vi "Periodic Tasks.vi"(8 "error in":errorcluster) -> ()   [LabVIEW 2014]
doc: "This VI runs in parallel to other tasks. It can contain as many user-defined periodic loops as you need. These can carry out PID or other sorts of timed response."
uses:
  NavX/navX-MXP Library/COMMON/TypeDefs/navX YPRH Data.ctl
  <vilib>/Rock Robotics/WPI/DriverStation/WPI_DriverStationRobotMode2.ctl
  <vilib>/Rock Robotics/WPI/Solenoid/WPI_SolenoidValue.ctl
  <vilib>/Rock Robotics/WPI/RobotDrive/WPI_RobotDriveGetSetRefNum.vi
  Robot Global Data.vi
  <vilib>/addons/control/pid/pid.llb/PID (DBL).vi
  <vilib>/Rock Robotics/WPI/RobotDrive/WPI_RobotDriveMecanumDrive_Cartesian.vi
  <vilib>/Rock Robotics/Network Tables/SD Write Numeric Array.vi
  <vilib>/Rock Robotics/Network Tables/SD Write Number.vi
  <vilib>/Rock Robotics/WPI/Joystick/WPI_JoystickGetSetRefNum.vi
  <vilib>/Rock Robotics/Network Tables/SD Write Boolean.vi
  <vilib>/Rock Robotics/Network Tables/SD Write String.vi
  <vilib>/Rock Robotics/WPI/Solenoid/WPI_SolenoidSetEnum.vi
  <vilib>/Rock Robotics/Network Tables/SD Read String.vi
  <vilib>/Utility/file.llb/Write To Spreadsheet File (DBL).vi
  <vilib>/addons/control/pid/pid.llb/PID Output Rate Limiter (DBL).vi
  NavX/navX-MXP Library/navX-MXP IMU.lvlib
  <vilib>/addons/control/pid/NI_PID_pid.lvlib
panel:
  in  "Turn PID Gains(Teley)":T1={"proportional gain (Kc)"=0.02, "integral time (Ti, min)"=0.0, "derivative time (Td, min)"=0.0}
  out "Angle":dbl
  out "Elevator Setpoint Limited":dbl
  out "Angle Data":T2(graph)
  in  "Manual Rate":dbl=30.0
  in  "Elevator PID gains (Seperation Corector)":T1={"proportional gain (Kc)"=0.007, "integral time (Ti, min)"=0.0, "derivative time (Td, min)"=0.0} {"derivative time (Td, min)" format="%.3f"; "integral time (Ti, min)" format="%.3f"; "proportional gain (Kc)" format="%.3f"}
  in  "Elevator Output Range (Seperation Corector)":cluster{"output high":dbl, "output low":dbl}={"output high"=0.25, "output low"=-0.1} {"output low" format="%.2f"; "output high" format="%.2f"}
  out "Encoder Ticks":i16
  in  "Elevator Output Range (RLPC/AVG)":cluster{"output high":dbl, "output low":dbl}={"output high"=1.0, "output low"=-0.5}
  out "Elevator Currents (A)":cluster{"current (A)":dbl, "current (A)":dbl}(graph)
  in  "output rate (EGU/min)":dbl=100000.0 format="%.2f"
  in  "Spin Cutoff":dbl=2.0
  in  "Elevator Cutoff Pos":dbl=20.0
  in  "Elevator PID Gains (RLPC/AVG)":T1={"proportional gain (Kc)"=0.003, "integral time (Ti, min)"=0.0, "derivative time (Td, min)"=0.0} {"proportional gain (Kc)" min=0.0 step=0.05 format="%.3f"; "integral time (Ti, min)" step=0.005 format="%.3f"; "derivative time (Td, min)" format="%.3f"}
  out "Elevator Setpoint":dbl
  in  "Turn PID Gains(Auto)":T1={"proportional gain (Kc)"=0.01, "integral time (Ti, min)"=0.016, "derivative time (Td, min)"=0.0} {"derivative time (Td, min)" format="%.3f"; "integral time (Ti, min)" format="%.3f"; "proportional gain (Kc)" format="%.3f"}
  out "Base PID Gains":T1={"proportional gain (Kc)"=1.0, "integral time (Ti, min)"=0.01, "derivative time (Td, min)"=0.0} {"derivative time (Td, min)" format="%.3f"; "integral time (Ti, min)" format="%.3f"; "proportional gain (Kc)" format="%.3f"}
  out "Spin Joy X":dbl
  in  "Use Knob?":bool=TRUE
  out "error out":errorcluster
  out "Y Setpoint":dbl
  out "X Setpoint":dbl
  out "Elevator Data":T3(graph)
  out "Closed Loop":bool
  out "Rear Right Distance":dbl
  out "Rear Left Distance":dbl
  out "Front Right Distance":dbl
  out "Front Left Distance":dbl
  out "Rear Right Rate":dbl(knob) scale=-1.0..1.0
  out "Rear Left Rate":dbl(knob) scale=-1.0..1.0
  out "Front Right Rate":dbl(knob) scale=-1.0..1.0
  out "Front Left Rate":dbl(knob) scale=-1.0..1.0
  out "appended array":dbl[](array[numeric])
  out "Angular Target":dbl
  out "YPRH":T4
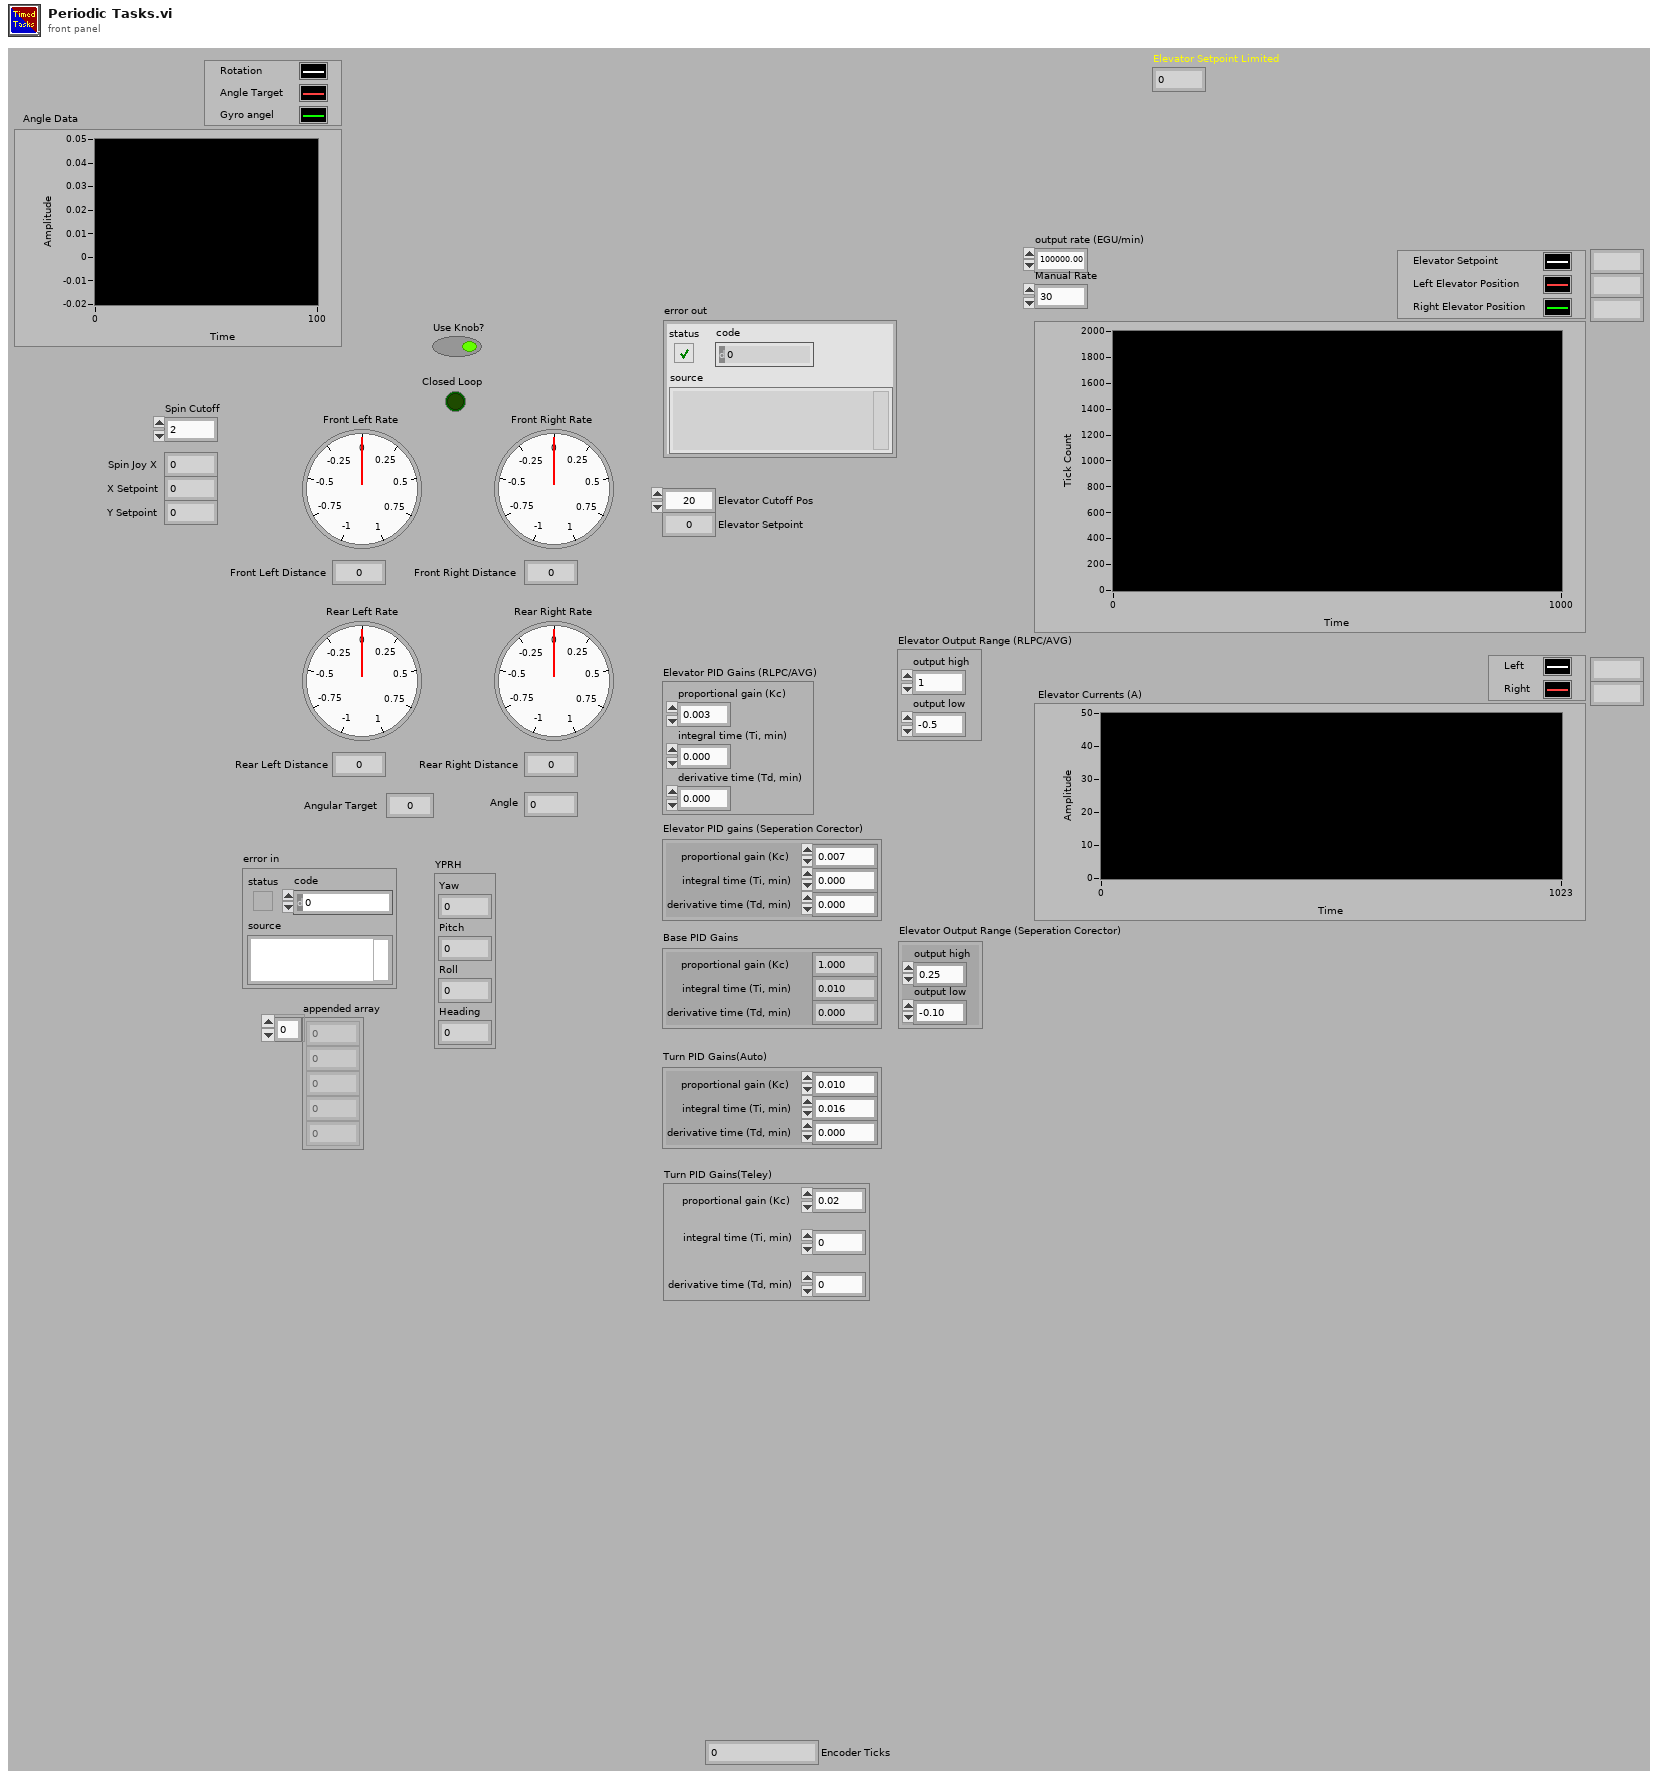
[diagram p1: front panel]
types:
  T1 = cluster{"proportional gain (Kc)":dbl, "integral time (Ti, min)":dbl, "derivative time (Td, min)":dbl}
  T2 = cluster{"t":dbl, "Angular Target":dbl, "Gyro Angle":dbl}
  T3 = cluster{"Elevator Setpoint":dbl, "Distance":dbl, "Distance":dbl}
  T4 = typedef "navX-MXP IMU.lvlib/navX YPRH Data.ctl" = cluster{"Yaw":dbl, "Pitch":dbl, "Roll":dbl, "Heading":dbl}
  T5 = typedef "WPI_EncoderDevRef.ctl" = cluster{"DevStatus":errorcluster, "EncoderIndex":T6, "CounterIndex":T7, "DistancePerCount":dbl, "Decoding Type":T8}
  T6 = typedef "FPGA_EncoderIdx.ctl" = enum8{"Enc 0", "Enc 1", "Enc 2", "Enc 3", "Enc 4", "Enc 5", "Enc 6", "Enc 7", "Invalid"}
  T7 = typedef "FPGA_CounterCtrSystemIndex.ctl" = enum8{"Ctr 0", "Ctr 1", "Ctr 2", "Ctr 3", "Ctr 4", "Ctr 5", "Ctr 6", "Ctr 7", "Invalid"}
  T8 = typedef "WPI_EncoderType.ctl" = enum16{"1x", "2x", "4x"}
  T9 = typedef "WPI_MotorControlDeviceRef.ctl" = cluster{"DeviceStatus":errorcluster, "Type":T10, "PWM":cluster{"Controller":T11, "PWM Channel":T12, "DeadBand":T13}, "CAN":cluster{"Device Number":u8, "Control Mode":T14, "Semaphore":T15, "Max Vout":dbl, "TalonSRX Control Mode":T16}, "Invert":bool, "TransformRef":T17, "InvTransformRef":T17}
  T10 = typedef "WPI_MotorControlType.ctl" = enum16{"PWM", "CAN", "CANTalonSRX"}
  T11 = typedef "FPGA_TypedefDigitalModule.ctl" = enum16{"Controller 1"}
  T12 = typedef "FPGA_DIOPWMChannel.ctl" = enum8{"PWM 0", "PWM 1", "PWM 2", "PWM 3", "PWM 4", "PWM 5", "PWM 6", "PWM 7", "PWM 8", "PWM 9", "PWM MXP 0", "PWM MXP 1", "PWM MXP 2", "PWM MXP 3", "PWM MXP 4", "PWM MXP 5", "PWM MXP 6", "PWM MXP 7", "PWM MXP 8", "PWM MXP 9", "Invalid"}
  T13 = typedef "WPI_PWMDeadband.ctl" = cluster{"Name":string, "maxPositivePwm":i32, "minPositivePwm":i32, "centerPwm":i32, "maxNegativePwm":i32, "minNegativePwm":i32, "angularRange":u16}
  T14 = typedef "WPI_CANJaguar_ControlMode.ctl" = enum8{"Percent VBus", "Current", "Speed", "Position", "Voltage"}
  T15 = typedef "Semaphore RefNum" = refnum<k1>
  T16 = typedef "WPI_CANTalonSRX_APIControlMode.ctl" = enum8{"Percent VBus", "Speed", "Position", "Slave", "Unchanged / Invalid"}
  T17 = typedef "WPI_PWMTransform_ConPane.ctl" = refnum<vi>
  T18 = typedef "WPI_DriverStationRobotMode2.ctl" = enum16{"Autonomous Disabled", "Autonomous Enabled", "Teleop Disabled", "Teleop Enabled", "Disconnected", "Finish", "Test Disabled", "Test Enabled", "Emergency Stopped"}
  T19 = cluster{"Elevator Setpoint Limited":dbl, "Distance":dbl, "Distance":dbl}
  T20 = typedef "navX-MXP IMU.lvlib/navX SPI DevRef.ctl" = cluster{"SPIDevRef":T21, "Board Information":T23, "Status":T24, "Offsets":cluster{"Yaw":dbl, "Quat W":dbl, "Quat X":dbl, "Quat Y":dbl, "Quat Z":dbl}, "Update Rate (4Hz-60Hz)":u8, "refnum name":string, "error":errorcluster}
  T21 = typedef "WPI_SPIDevRef.ctl" = cluster{"DevStatus":errorcluster, "Handle":i32, "Controller":T11, "SPI Bus":T22}
  T22 = typedef "spi_bus.ctl" = enum16{"SPI On-Board, CS0", "SPI On-Board, CS1", "SPI On-Board, CS2", "SPI On-Board, CS3", "SPI MXP", "Invalid"}
  T23 = typedef "navX-MXP IMU.lvlib/navX Board Information.ctl" = cluster{"WhoAmI (50 | 0x32)":u8, "Board Revision":u8, "Firmware Major Version":u8, "Firmware Minor Version":u8}
  T24 = typedef "navX-MXP IMU.lvlib/navX Status Data.ctl" = cluster{"Update Rate Hz":u8, "Accelerometer Full-Scale Range":u8, "Gyro Full-Scale Range":u16, "NAVX_OP_STATUS":T25, "NAVX_CAL_STATUS":T26, "NAVX_SELFTEST_STATUS":u8, "NAVX_SENSOR_STATUS":T27}
  T25 = typedef "navX-MXP IMU.lvlib/navX NAVX_OP_STATUS.ctl" = u8
  T26 = typedef "navX-MXP IMU.lvlib/navX NAVX_CAL_STATUS.ctl" = u8
  T27 = typedef "navX-MXP IMU.lvlib/navX NAVX_SENSOR_STATUS.ctl" = cluster{"MOVING":bool, "YAW_STABLE":bool, "MAG_DISTURBANCE":bool, "ALTITUDE_VALID":bool, "SEALEVEL_PRESS_SET":bool, "FUSED_HEADING_VALID":bool}
  T28 = typedef "WPI_RobotDriveDevRef.ctl" = cluster{"DevStatus":errorcluster, "Motors[]":T9[], "Square Inputs":bool, "Max Output":dbl}
  T29 = typedef "WPI_GyroDevRef.ctl" = cluster{"DevStatus":errorcluster, "Analog Module":T30, "Analog Channel":T31, "Offset":dbl, "Gain (VoltsPerDegree/Second)":dbl}
  T30 = typedef "FPGA_TypedefAnalogModule.ctl" = enum16{"Controller 1"}
  T31 = typedef "FPGA_AIChannel.ctl" = enum8{"AI 0", "AI 1", "AI 2", "AI 3", "AI MXP 0", "AI MXP 1", "AI MXP 2", "AI MXP 3", "Invalid"}
  T32 = typedef "WPI_SolenoidDevRef.ctl" = cluster{"DevStatus":errorcluster, "Pneumatics Control Module":u8, "Forward Solenoid Channel":T33, "Reverse Solenoid Channel":T33}
  T33 = typedef "WPI_SolenoidChannel.ctl" = enum8{"Solenoid 0", "Solenoid 1", "Solenoid 2", "Solenoid 3", "Solenoid 4", "Solenoid 5", "Solenoid 6", "Solenoid 7", "Invalid"}
  T34 = typedef "WPI_JoystickDevRef.ctl" = cluster{"Device":T35}
  T35 = typedef "WPI_JoystickDeviceEnum.ctl" = enum16{"USB 0", "USB 1", "USB 2", "USB 3", "USB 4", "USB 5"}
  T36 = typedef "WPI_SolenoidValue.ctl" = enum16{"Off", "On", "Forward", "Reverse"}
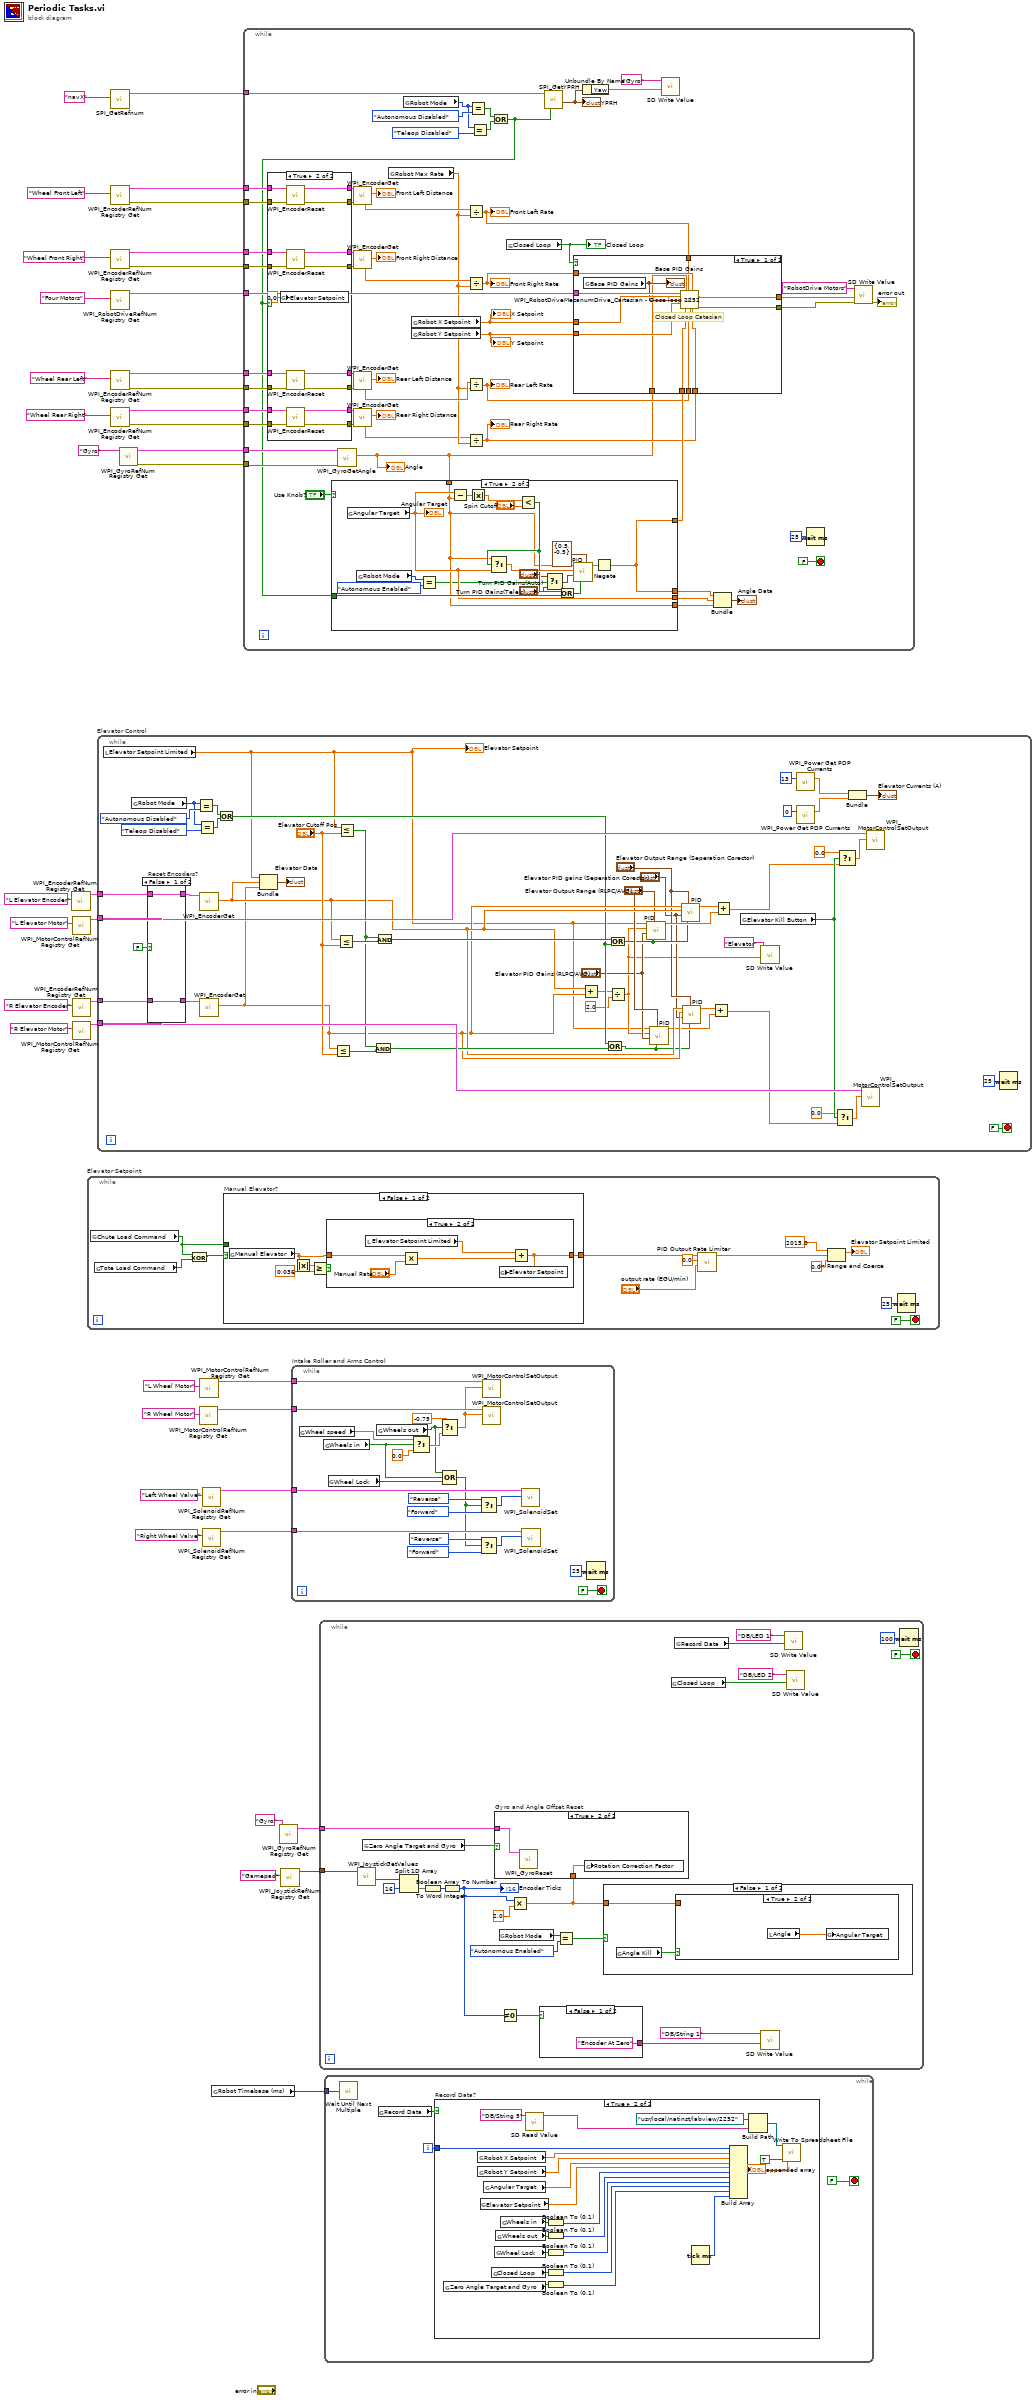
[diagram p0: block diagram]
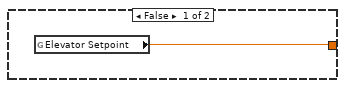
[diagram p2: hidden frame]
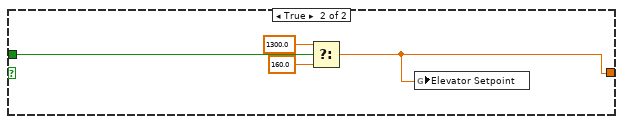
[diagram p3: hidden frame]
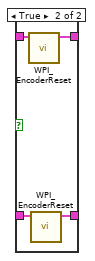
[diagram p4: hidden frame]
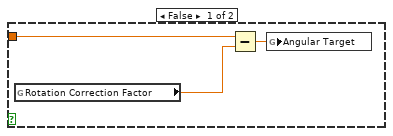
[diagram p5: hidden frame]
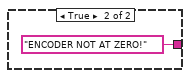
[diagram p7: hidden frame]
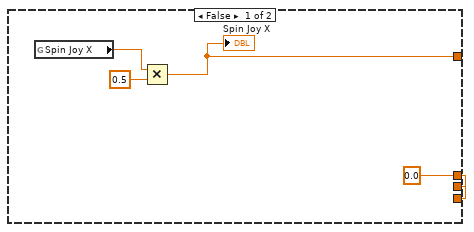
[diagram p11: hidden frame]
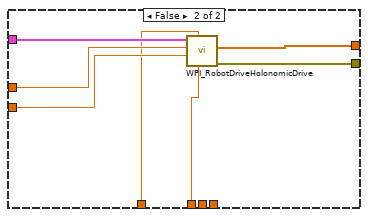
[diagram p12: hidden frame]
diagram:
  n1 = call <vilib>:"WPI_EncoderRefNum Registry Get.vi"("refnum name"="L Elevator Encoder") -> ("EncoderDevRef"=w19:T5)  [unwired: 9 in, 1 out]
  n2 = call <vilib>:"WPI_MotorControlRefNum Registry Get.vi"("refnum name"="L Elevator Motor") -> ("MotorControlDevRef"=w13:T9)  [unwired: 9 in, 1 out]
  n3 = call <vilib>:"WPI_EncoderRefNum Registry Get.vi"("refnum name"="R Elevator Encoder") -> ("EncoderDevRef"=w18:T5)  [unwired: 9 in, 1 out]
  n4 = call <vilib>:"WPI_MotorControlRefNum Registry Get.vi"("refnum name"="R Elevator Motor") -> ("MotorControlDevRef"=w14:T9)  [unwired: 9 in, 1 out]
  n5 = while "Elevator Setpoint" {
    stop <- FALSE stop-if-true
    n6 = global read "Robot Global Data.vi" "Chute Load Command"() -> (w42:bool)
    n7 = global read "Robot Global Data.vi" "Tote Load Command"() -> (w43:bool)
    n8 = Exclusive Or(1:w43, 2:w42) -> (0:w44:bool)
    n9 = case "Manual Elevator?" shown="False" w44 {
      tunnel: [w57 w64] -> w48
      tunnel: w42 -> [_ w67]
      frame False {
        n10 = global read "Robot Global Data.vi" "Manual Elevator"() -> (w54:dbl)
        n11 = Absolute Value(x=w54) -> (abs(x)=w53:dbl)
        n12 = Greater Or Equal?(x=w53, y=0.036) -> (x >= y?=w55:bool)
        n13 = case shown="True" w55 {
          tunnel: w54 -> [_ w62]
          tunnel: [w58 w59] -> w57
          frame False {
            n14 = global read "Robot Global Data.vi" "Elevator Setpoint"() -> (w58:dbl)
          }
          frame True {
            n15 = local read "Elevator Setpoint Limited"() -> (w60:dbl)
            n16 = Multiply(x=w62, y="Manual Rate") -> (x*y=w63:dbl)
            n17 = Add(x=w60, y=w63) -> (x+y=w59:dbl)
            n18 = global write "Robot Global Data.vi" "Elevator Setpoint"(w59) -> ()
          }
        }
      }
      frame True {
        n19 = Select(t=1300.0, s=w67, f=160.0) -> (s? t:f=w64:dbl)
        n20 = global write "Robot Global Data.vi" "Elevator Setpoint"(w64) -> ()
      }
    }
    n21 = call-poly <vilib>:"PID Output Rate Limiter.vi"("output rate (EGU/min)"="output rate (EGU/min)", "initial output"=0.0, "input (controller output)"=w48) -> ("output"=w49:dbl)  [unwired: 5 in, 1 out]
    n22 = In Range and Coerce(upper limit=2015.0, x=w49, lower limit=0.0) -> (coerced(x)=→"Elevator Setpoint Limited":dbl)  [unwired: 1 out]
    n23 = Wait (ms)(milliseconds to wait=u32 25) -> ()  [unwired: 1 out]
  }
  n24 = while "Elevator Control" {
    tunnel: w19 -> [w104]
    tunnel: w18 -> [w105]
    tunnel: w14 -> [w117]
    tunnel: w13 -> [w116]
    stop <- FALSE stop-if-true
    n25 = local read "Elevator Setpoint Limited"() -> (w76:dbl)
    "Elevator Setpoint" <- w76
    n26 = global read "Robot Global Data.vi" "Robot Mode"() -> (w97:T18)
    n27 = case "Reset Encoders?" shown="False" FALSE {
      tunnel: w105 -> [w120 w124]
      tunnel: w104 -> [w119 w123]
      tunnel: [w119 w122] -> w103
      tunnel: [w120 w121] -> w102
      frame False {
      }
      frame True {
        n28 = call <vilib>:"WPI_EncoderReset.vi"("EncoderDevRef"=w123) -> ("EncoderDevRef"=w122:T5)  [unwired: 9 in, 1 out]
        n29 = call <vilib>:"WPI_EncoderReset.vi"("EncoderDevRef"=w124) -> ("EncoderDevRef"=w121:T5)  [unwired: 9 in, 1 out]
      }
    }
    n30 = Equal?(x=w97, y=WPI_DriverStationRobotMode2."Autonomous Disabled") -> (x = y?=w100:bool)
    n31 = Equal?(x=w97, y=WPI_DriverStationRobotMode2."Teleop Disabled") -> (x = y?=w99:bool)
    n32 = call <vilib>:"WPI_EncoderGet.vi"("EncoderDevRef"=w103) -> ("Distance"=w107:dbl)  [unwired: 5 in, 5 out]
    n33 = call <vilib>:"WPI_EncoderGet.vi"("EncoderDevRef"=w102) -> ("Distance"=w106:dbl)  [unwired: 5 in, 5 out]
    n34 = Or(x=w100, y=w99) -> (x .or. y?=w98:bool)
    n35 = Bundle("Elevator Setpoint Limited"=w76, "Distance"=w107, "Distance"=w106) -> (→"Elevator Data":T19)  [unwired: 1 in]
    n36 = Less Or Equal?(x=w106, y="Elevator Cutoff Pos") -> (x <= y?=w115:bool)
    n37 = Less Or Equal?(x=w107, y="Elevator Cutoff Pos") -> (x <= y?=w114:bool)
    n38 = Less Or Equal?(x=w76, y="Elevator Cutoff Pos") -> (x <= y?=w112:bool)
    n39 = And(x=w112, y=w115) -> (x .and. y?=w110:bool)
    n40 = And(x=w112, y=w114) -> (x .and. y?=w109:bool)
    n41 = Add(x=w107, y=w106) -> (x+y=w83:dbl)
    n42 = Or(x=w98, y=w110) -> (x .or. y?=w85:bool)
    n43 = Or(x=w109, y=w98) -> (x .or. y?=w84:bool)
    n44 = Divide(x=w83, y=2.0) -> (x/y=w77:dbl)
    n45 = call-poly <vilib>:"PID.vi"("reinitialize? (F)"=w84, "output range"="Elevator Output Range (RLPC/AVG)", "PID gains"="Elevator PID Gains (RLPC/AVG)", "process variable"=w77, "setpoint"=w76) -> ("output"=w89:dbl)  [unwired: 5 in, 1 out]
    n46 = call-poly <vilib>:"PID.vi"("reinitialize? (F)"=w85, "output range"="Elevator Output Range (RLPC/AVG)", "PID gains"="Elevator PID Gains (RLPC/AVG)", "process variable"=w77, "setpoint"=w76) -> ("output"=w87:dbl)  [unwired: 5 in, 1 out]
    n47 = call-poly <vilib>:"PID.vi"("reinitialize? (F)"=w84, "output range"="Elevator Output Range (Seperation Corector)", "PID gains"="Elevator PID gains (Seperation Corector)", "process variable"=w107, "setpoint"=w106) -> ("output"=w88:dbl)  [unwired: 5 in, 1 out]
    n48 = call-poly <vilib>:"PID.vi"("reinitialize? (F)"=w85, "output range"="Elevator Output Range (Seperation Corector)", "PID gains"="Elevator PID gains (Seperation Corector)", "process variable"=w106, "setpoint"=w107) -> ("output"=w86:dbl)  [unwired: 5 in, 1 out]
    n49 = Add(x=w86, y=w87) -> (x+y=w69:dbl)
    n50 = Add(x=w88, y=w89) -> (x+y=w72:dbl)
    n51 = global read "Robot Global Data.vi" "Elevator Kill Button"() -> (w73:bool)
    n52 = call-poly <vilib>:"SD Write Value.vi"("Numeric"=w77, "Name"="Elevator") -> ()  [unwired: 8 in, 2 out]
    n53 = call <vilib>:"WPI_Power Get PDP Currents.vi"("PDP Channel"=13) -> ("current (A)"=w92:dbl)  [unwired: 12 in, 2 out]
    n54 = call <vilib>:"WPI_Power Get PDP Currents.vi"("PDP Channel"=0) -> ("current (A)"=w91:dbl)  [unwired: 12 in, 2 out]
    n55 = Select(t=0.0 ("f"), s=w73, f=w69) -> (s? t:f=w74:dbl)
    n56 = Select(t=0.0, s=w73, f=w72) -> (s? t:f=w75:dbl)
    n57 = Bundle("current (A)"=w92, "current (A)"=w91) -> (→"Elevator Currents (A)":cluster{"current (A)":dbl, "current (A)":dbl})  [unwired: 1 in]
    n58 = call <vilib>:"WPI_MotorControlSetOutput.vi"("Output"=w74, "MotorControlDevRef"=w117) -> ()  [unwired: 7 in, 3 out]
    n59 = call <vilib>:"WPI_MotorControlSetOutput.vi"("Output"=w75, "MotorControlDevRef"=w116) -> ()  [unwired: 7 in, 3 out]
    n60 = Wait (ms)(milliseconds to wait=u32 25) -> ()  [unwired: 1 out]
  }
  n61 = call "SPI_GetRefnum.vi"("refnum name"="navX") -> ("navX DevRef"=w39:T20)  [unwired: 9 in, 1 out]
  n62 = call <vilib>:"WPI_EncoderRefNum Registry Get.vi"("refnum name"="Wheel Front Left") -> ("error out"=w25:errorcluster, "EncoderDevRef"=w33:T5)  [unwired: 9 in]
  n63 = call <vilib>:"WPI_EncoderRefNum Registry Get.vi"("refnum name"="Wheel Front Right") -> ("error out"=w24:errorcluster, "EncoderDevRef"=w30:T5)  [unwired: 9 in]
  n64 = call <vilib>:"WPI_RobotDriveRefNum Registry Get.vi"("refnum name"="Four Motors") -> ("RobotDriveDevRef"=w35:T28)  [unwired: 1 in, 9 out]
  n65 = call <vilib>:"WPI_EncoderRefNum Registry Get.vi"("refnum name"="Wheel Rear Left") -> ("error out"=w23:errorcluster, "EncoderDevRef"=w29:T5)  [unwired: 9 in]
  n66 = call <vilib>:"WPI_EncoderRefNum Registry Get.vi"("refnum name"="Wheel Rear Right") -> ("error out"=w22:errorcluster, "EncoderDevRef"=w26:T5)  [unwired: 9 in]
  n67 = call <vilib>:"WPI_GyroRefNum Registry Get.vi"("refnum name"="Gyro") -> ("error out"=w21:errorcluster, "GyroDevRef"=w37:T29)  [unwired: 9 in]
  n68 = call <vilib>:"WPI_MotorControlRefNum Registry Get.vi"("refnum name"="R Wheel Motor") -> ("MotorControlDevRef"=w11:T9)  [unwired: 9 in, 1 out]
  n69 = call <vilib>:"WPI_MotorControlRefNum Registry Get.vi"("refnum name"="L Wheel Motor") -> ("MotorControlDevRef"=w12:T9)  [unwired: 9 in, 1 out]
  n70 = call <vilib>:"WPI_SolenoidRefNum Registry Get.vi"("refnum name"="Left Wheel Valve") -> ("SolenoidDevRef"=w2:T32)  [unwired: 9 in, 1 out]
  n71 = call <vilib>:"WPI_SolenoidRefNum Registry Get.vi"("refnum name"="Right Wheel Valve") -> ("SolenoidDevRef"=w1:T32)  [unwired: 9 in, 1 out]
  n72 = global read "Robot Global Data.vi" "Robot Timebase (ms)"() -> (w34:u32)
  n73 = while {
    tunnel: w39 -> [w180]
    tunnel: w37 -> [w173]
    tunnel: w35 -> [w171]
    tunnel: w33 -> [w134]
    tunnel: w30 -> [w136]
    tunnel: w29 -> [w138]
    tunnel: w26 -> [w140]
    tunnel: w25 -> [w142]
    tunnel: w24 -> [w144]
    tunnel: w23 -> [w146]
    tunnel: w22 -> [w148]
    tunnel: w21 -> [w167]
    stop <- FALSE stop-if-true
    n74 = call <vilib>:"WPI_GyroGetAngle.vi"("error in (no error)"=w167, "GyroDevRef"=w173) -> ("Angle"=w126:dbl)  [unwired: 6 in, 3 out]
    "Angle" <- w126
    n75 = global read "Robot Global Data.vi" "Robot Max Rate"() -> (w151:dbl)
    n76 = global read "Robot Global Data.vi" "Robot Mode"() -> (w175:T18)
    n77 = global read "Robot Global Data.vi" "Robot X Setpoint"() -> (w154:dbl)
    "X Setpoint" <- w154
    n78 = global read "Robot Global Data.vi" "Robot Y Setpoint"() -> (w155:dbl)
    "Y Setpoint" <- w155
    n79 = Equal?(x=w175, y=WPI_DriverStationRobotMode2."Autonomous Disabled") -> (x = y?=w178:bool)
    n80 = Equal?(x=w175, y=WPI_DriverStationRobotMode2."Teleop Disabled") -> (x = y?=w176:bool)
    n81 = Or(x=w178, y=w176) -> (x .or. y?=w131:bool)
    n82 = case shown="True" w131 {
      tunnel: w148 -> [w183 w207]
      tunnel: [w183 w206] -> w147
      tunnel: w146 -> [w185 w205]
      tunnel: [w185 w204] -> w145
      tunnel: w144 -> [w187 w203]
      tunnel: [w187 w202] -> w143
      tunnel: w142 -> [w189 w201]
      tunnel: [w189 w200] -> w141
      tunnel: w140 -> [w184 w199]
      tunnel: [w184 w198] -> w139
      tunnel: w138 -> [w186 w197]
      tunnel: [w186 w196] -> w137
      tunnel: w136 -> [w188 w195]
      tunnel: [w188 w194] -> w135
      tunnel: w134 -> [w190 w193]
      tunnel: [w190 w192] -> w133
      frame False {
      }
      frame True {
        n83 = global write "Robot Global Data.vi" "Elevator Setpoint"(0.0 ("Elevator Setpoint")) -> ()
        n84 = call <vilib>:"WPI_EncoderReset.vi"("error in (no error)"=w201, "EncoderDevRef"=w193) -> ("error out"=w200:errorcluster, "EncoderDevRef"=w192:T5)  [unwired: 8 in]
        n85 = call <vilib>:"WPI_EncoderReset.vi"("error in (no error)"=w203, "EncoderDevRef"=w195) -> ("error out"=w202:errorcluster, "EncoderDevRef"=w194:T5)  [unwired: 8 in]
        n86 = call <vilib>:"WPI_EncoderReset.vi"("error in (no error)"=w205, "EncoderDevRef"=w197) -> ("error out"=w204:errorcluster, "EncoderDevRef"=w196:T5)  [unwired: 8 in]
        n87 = call <vilib>:"WPI_EncoderReset.vi"("error in (no error)"=w207, "EncoderDevRef"=w199) -> ("error out"=w206:errorcluster, "EncoderDevRef"=w198:T5)  [unwired: 8 in]
      }
    }
    n88 = case shown="True" "Use Knob?" {
      tunnel: [w209 w220] -> w170
      tunnel: w126 -> [_ w218]
      tunnel: w131 -> [_ w223]
      tunnel: [w208 w220] -> w129
      tunnel: [w208 w219] -> w128
      tunnel: [w208 w218] -> w127
      frame False {
        w208 = 0.0
        n89 = global read "Robot Global Data.vi" "Spin Joy X"() -> (w210:dbl)
        n90 = Multiply(x=w210, y=0.5) -> (x*y=w209:dbl)
        "Spin Joy X" <- w209
      }
      frame True {
        n91 = global read "Robot Global Data.vi" "Angular Target"() -> (w219:dbl)
        "Angular Target" <- w219
        n92 = global read "Robot Global Data.vi" "Robot Mode"() -> (w214:T18)
        n93 = Equal?(x=w214, y=WPI_DriverStationRobotMode2."Autonomous Enabled") -> (x = y?=w212:bool)
        n94 = Subtract(x=w219, y=w218) -> (x-y=w227:dbl)
        n95 = Absolute Value(x=w227) -> (abs(x)=w226:dbl)
        n96 = Less?(x=w226, y="Spin Cutoff") -> (x < y?=w221:bool)
        n97 = Select(t=w218, s=w221, f=w219) -> (s? t:f=w222:dbl)
        n98 = Select(t="Turn PID Gains(Auto)", s=w212, f="Turn PID Gains(Teley)") -> (s? t:f=w216:T1)
        n99 = Or(x=w221, y=w223) -> (x .or. y?=w224:bool)
        n100 = call-poly <vilib>:"PID.vi"("reinitialize? (F)"=w224, "output range"=cluster{"output high":dbl, "output low":dbl} {"output high"=0.5, "output low"=-0.5}, "PID gains"=w216, "process variable"=w222, "setpoint"=w218) -> ("output"=w228:dbl)  [unwired: 5 in, 1 out]
        n101 = Negate(x=w228) -> (-x=w220:dbl)
      }
    }
    n102 = call <vilib>:"WPI_EncoderGet.vi"("error in (no error)"=w141, "EncoderDevRef"=w133) -> ("Distance"=→"Front Left Distance":dbl, "Rate"=w159:dbl)  [unwired: 4 in, 4 out]
    n103 = call <vilib>:"WPI_EncoderGet.vi"("error in (no error)"=w143, "EncoderDevRef"=w135) -> ("Distance"=→"Front Right Distance":dbl, "Rate"=w157:dbl)  [unwired: 4 in, 4 out]
    n104 = call <vilib>:"WPI_EncoderGet.vi"("error in (no error)"=w145, "EncoderDevRef"=w137) -> ("Distance"=→"Rear Left Distance":dbl, "Rate"=w153:dbl)  [unwired: 4 in, 4 out]
    n105 = call <vilib>:"WPI_EncoderGet.vi"("error in (no error)"=w147, "EncoderDevRef"=w139) -> ("Distance"=→"Rear Right Distance":dbl, "Rate"=w150:dbl)  [unwired: 4 in, 4 out]
    n106 = Divide(x=w159, y=w151) -> (x/y=w158:dbl)
    "Front Left Rate" <- w158
    n107 = Divide(x=w157, y=w151) -> (x/y=w156:dbl)
    "Front Right Rate" <- w156
    n108 = Divide(x=w153, y=w151) -> (x/y=w152:dbl)
    "Rear Left Rate" <- w152
    n109 = Divide(x=w150, y=w151) -> (x/y=w149:dbl)
    "Rear Right Rate" <- w149
    n110 = global read "Robot Global Data.vi" "Closed Loop"() -> (w168:bool)
    "Closed Loop" <- w168
    n111 = call "SPI_GetYPRH.vi"("Zero"=w131, "navX DevRef"=w180) -> ("YPRH"=w174:T4)  [unwired: 7 in, 2 out]
    "YPRH" <- w174
    n112 = case shown="True" w168 {
      tunnel: w171 -> [w241 w248]
      tunnel: w155 -> [w239 w247]
      tunnel: w154 -> [w240 w246]
      tunnel: w170 -> [w232 w245]
      tunnel: [w234 w244] -> w169
      tunnel: w158 -> [w236 _]
      tunnel: w156 -> [w237 _]
      tunnel: w149 -> [w230 _]
      tunnel: w152 -> [w231 _]
      tunnel: w126 -> [w235 w243]
      tunnel: [w233 w242] -> w161
      frame True {
        # "Closed Loop Catesian"
        n113 = global read "Robot Global Data.vi" "Base PID Gains"() -> (w238:T1)
        "Base PID Gains" <- w238
        n114 = call "WPI_RobotDriveMecanumDrive_Cartesian - Close loop 2252.vi"("RobotDriveDevRef"=w241, "Gyro Angle"=w235, "Encoder Front Left"=w236, "Encoder Front Right"=w237, "X (-1 to 1)"=w240, "PID gains"=w238, "Y (-1 to 1)"=w239, "Rotation"=w232, "Encoder Rear Left"=w231, "Encoder Rear Right"=w230) -> ("Motor Values"=w234:dbl[], "error out"=w233:errorcluster)  [unwired: 3 in, 1 out]
      }
      frame False {
        n115 = call-poly <vilib>:"WPI_RobotDriveHolonomicDrive.vi"("Rotation"=w245, "Gyro Angle"=w243, "Y"=w247, "X"=w246, "RobotDriveDevRef"=w248) -> ("error out"=w242:errorcluster, "Motor Values"=w244:dbl[])  [unwired: 4 in, 1 out]
      }
    }
    n116 = Unbundle By Name(w174) -> ("Yaw"=w132:dbl)
    n117 = call-poly <vilib>:"SD Write Value.vi"("Numeric"=w132, "Name"="Gyro") -> ()  [unwired: 8 in, 2 out]
    n118 = Bundle(w129, "Angular Target"=w128, "Angle"=w127) -> (→"Angle Data":cluster{dbl, "Angular Target":dbl, "Angle":dbl})  [unwired: 1 in]
    n119 = Wait (ms)(milliseconds to wait=u32 25) -> ()  [unwired: 1 out]
    n120 = call-poly <vilib>:"SD Write Value.vi"("error in"=w161, "Numeric Array"=w169, "Name"="RobotDrive Motors") -> ("error out"=→"error out":errorcluster)  [unwired: 7 in, 1 out]
  }
  n121 = call <vilib>:"WPI_GyroRefNum Registry Get.vi"("refnum name"="Gyro") -> ("GyroDevRef"=w5:T29)  [unwired: 9 in, 1 out]
  n122 = call <vilib>:"WPI_JoystickRefNum Registry Get.vi"("refnum name"="Gamepad") -> ("JoystickDevRef"=w7:T34)  [unwired: 1 in, 9 out]
  n123 = while "Intake Roller and Arms Control" {
    tunnel: w12 -> [w267]
    tunnel: w11 -> [w266]
    tunnel: w2 -> [w257]
    tunnel: w1 -> [w255]
    stop <- FALSE stop-if-true
    n124 = global read "Robot Global Data.vi" "Wheel speed"() -> (w262:dbl)
    n125 = global read "Robot Global Data.vi" "Wheels in"() -> (w251:bool)
    n126 = global read "Robot Global Data.vi" "Wheel Lock"() -> (w250:bool)
    n127 = global read "Robot Global Data.vi" "Wheels out"() -> (w252:bool)
    n128 = Select(t=w262, s=w251, f=0.0) -> (s? t:f=w264:dbl)
    n129 = Select(t=-0.75, s=w252, f=w264) -> (s? t:f=w265:dbl)
    n130 = Compound Arithmetic op=OR(w252, w251, w250) -> (w253:bool)
    n131 = Select(t=WPI_SolenoidValue."Reverse" ("Value"), s=w253, f=WPI_SolenoidValue."Forward" ("Value")) -> (s? t:f=w256:T36)
    n132 = Select(t=WPI_SolenoidValue."Reverse" ("Value"), s=w253, f=WPI_SolenoidValue."Forward" ("Value")) -> (s? t:f=w254:T36)
    n133 = call <vilib>:"WPI_MotorControlSetOutput.vi"("Output"=w265, "MotorControlDevRef"=w267) -> ()  [unwired: 7 in, 3 out]
    n134 = call <vilib>:"WPI_MotorControlSetOutput.vi"("Output"=w265, "MotorControlDevRef"=w266) -> ()  [unwired: 7 in, 3 out]
    n135 = call-poly <vilib>:"WPI_SolenoidSet.vi"("Value"=w256, "SolenoidDevRef"=w257) -> ()  [unwired: 8 in, 2 out]
    n136 = call-poly <vilib>:"WPI_SolenoidSet.vi"("Value"=w254, "SolenoidDevRef"=w255) -> ()  [unwired: 8 in, 2 out]
    n137 = Wait (ms)(milliseconds to wait=u32 25) -> ()  [unwired: 1 out]
  }
  n138 = while {
    tunnel: w7 -> [w279]
    tunnel: w5 -> [w277]
    stop <- FALSE stop-if-true
    n139 = call <vilib>:"WPI_JoystickGetValues.vi"("JoystickDevRef"=w279) -> ("Buttons"=w281:bool[])  [unwired: 6 in, 4 out]
    n140 = global read "Robot Global Data.vi" "Zero Angle Target and Gyro"() -> (w278:bool)
    n141 = Split 1D Array(array=w281, index=16) -> (second subarray=w283:bool[])  [unwired: 1 out]
    n142 = Boolean Array To Number(Boolean array=w283) -> (number=w284:u32)
    n143 = To Word Integer(number=w284) -> (16bit integer=w273:i16)
    "Encoder Ticks" <- w273
    n144 = global read "Robot Global Data.vi" "Robot Mode"() -> (w272:T18)
    n145 = Not Equal To 0?(x=w273) -> (x != 0?=w274:bool)
    n146 = Multiply(x=w273, y=2.0) -> (x*y=w285:dbl)
    n147 = case "Gyro and Angle Offset Reset" shown="True" w278 {
      tunnel: w285 -> [_ w301]
      tunnel: w277 -> [_ w300]
      frame False {
      }
      frame True {
        n148 = call <vilib>:"WPI_GyroReset.vi"("GyroDevRef"=w300) -> ()  [unwired: 9 in, 2 out]
        n149 = global write "Robot Global Data.vi" "Rotation Correction Factor"(w301) -> ()
      }
    }
    n150 = case shown="False" w274 {
      tunnel: ["Encoder At Zero" ("String") "ENCODER NOT AT ZERO!" ("String")] -> w275
      frame False {
      }
      frame True {
      }
    }
    n151 = Equal?(x=w272, y=WPI_DriverStationRobotMode2."Autonomous Enabled") -> (x = y?=w270:bool)
    n152 = case shown="False" w270 {
      tunnel: w285 -> [w293 _]
      frame False {
        n153 = global read "Robot Global Data.vi" "Angle Kill"() -> (w292:bool)
        n154 = case shown="True" w292 {
          tunnel: w293 -> [w296 _]
          frame False {
            n155 = global read "Robot Global Data.vi" "Rotation Correction Factor"() -> (w295:dbl)
            n156 = Subtract(x=w296, y=w295) -> (x-y=w294:dbl)
            n157 = global write "Robot Global Data.vi" "Angular Target"(w294) -> ()
          }
          frame True {
            n158 = local read "Angle"() -> (w297:dbl)
            n159 = global write "Robot Global Data.vi" "Angular Target"(w297) -> ()
          }
        }
      }
      frame True {
      }
    }
    n160 = global read "Robot Global Data.vi" "Closed Loop"() -> (w287:bool)
    n161 = global read "Robot Global Data.vi" "Record Data"() -> (w288:bool)
    n162 = call-poly <vilib>:"SD Write Value.vi"("String"=w275, "Name"="DB/String 1") -> ()  [unwired: 8 in, 2 out]
    n163 = call-poly <vilib>:"SD Write Value.vi"("Boolean"=w288, "Name"="DB/LED 1") -> ()  [unwired: 8 in, 2 out]
    n164 = call-poly <vilib>:"SD Write Value.vi"("Boolean"=w287, "Name"="DB/LED 2") -> ()  [unwired: 8 in, 2 out]
    n165 = Wait (ms)(milliseconds to wait=u32 100) -> ()  [unwired: 1 out]
  }
  n166 = while {
    tunnel: w34 -> [w303]
    i -> [w304]
    stop <- FALSE stop-if-true
    n167 = call "Wait Until Next Multiple"("Count(mSec)"=w303) -> ()  [unwired: 1 out]
    n168 = global read "Robot Global Data.vi" "Record Data"() -> (w302:bool)
    n169 = case "Record Data?" shown="True" w302 {
      tunnel: w304 -> [_ w326]
      frame False {
      }
      frame True {
        n170 = global read "Robot Global Data.vi" "Zero Angle Target and Gyro"() -> (w313:bool)
        n171 = global read "Robot Global Data.vi" "Robot X Setpoint"() -> (w318:dbl)
        n172 = global read "Robot Global Data.vi" "Robot Y Setpoint"() -> (w319:dbl)
        n173 = global read "Robot Global Data.vi" "Elevator Setpoint"() -> (w308:dbl)
        n174 = global read "Robot Global Data.vi" "Angular Target"() -> (w320:dbl)
        n175 = global read "Robot Global Data.vi" "Closed Loop"() -> (w314:bool)
        n176 = global read "Robot Global Data.vi" "Wheel Lock"() -> (w307:bool)
        n177 = global read "Robot Global Data.vi" "Wheels out"() -> (w315:bool)
        n178 = global read "Robot Global Data.vi" "Wheels in"() -> (w316:bool)
        n179 = call-poly <vilib>:"SD Read Value.vi"("Name"="DB/String 5") -> ("String"=w322:string)  [unwired: 8 in, 2 out]
        n180 = Boolean To (0,1)(Boolean=w316) -> (0, 1=w312:i16)
        n181 = Boolean To (0,1)(Boolean=w315) -> (0, 1=w311:i16)
        n182 = Boolean To (0,1)(Boolean=w307) -> (0, 1=w306:i16)
        n183 = Boolean To (0,1)(Boolean=w314) -> (0, 1=w310:i16)
        n184 = Boolean To (0,1)(Boolean=w313) -> (0, 1=w309:i16)
        n185 = Tick Count (ms)() -> (millisecond timer value=w317:u32)
        n186 = Build Array(w326, w318, w319, w320, w308, w312, w311, w306, w310, w309, w317) -> (w327:dbl[])
        "appended array" <- w327
        n187 = Build Path(base path=path "/usr/local/natinst/labview/2252", name or relative path=w322) -> (appended path=w324:path)
        n188 = call-poly <vilib>:"Write To Spreadsheet File.vi"("append to file? (new file:F)"=TRUE, "1D data"=w327, "file path (dialog if empty)"=w324) -> ()  [unwired: 3 in, 3 out]
      }
    }
  }
